vi "PNDT-Draw Line.vi"(0 "picture":picture, 2 "end point":cluster{"x":i16, "y":i16}, 3 "absolute coordinates?(T)":bool=TRUE, 4 "pen":T1={"Lable"="", "Visible"=FALSE, "Width"=1, "Colour"=10263708, "Line"=enum."DashDotDot"} {"Width" min=1 max=5}) -> (6 "new picture":picture)   [LabVIEW 2026, in "MicroPulse_Driver.lvlib"]
doc: "Draws a line from the current pen position to the specified location in a picture."
uses:
  MicroPulse_Driver.lvlib
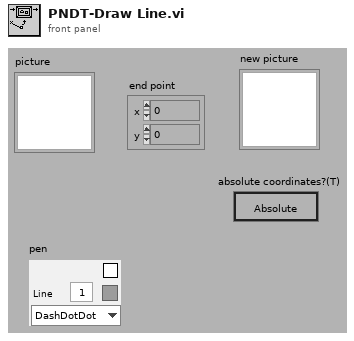
[diagram p1: front panel]
types:
  T1 = cluster{"Lable":string, "Visible":bool, "Width":u16, "Colour":u32, "Line":enum32{"Solid", "Dash", "Dot", "DashDot", "DashDotDot"}}
  T2 = enum32{"Solid", "Dash", "Dot", "DashDot", "DashDotDot"}
  T3 = cluster{"opcode-Select Pen":i16, "size":i32, "PictPen ID":i32, "pen mask":i32, "Colour":u32, "Width":u16, "Line":enum32{"Solid", "Dash", "Dot", "DashDot", "DashDotDot"}}
  T4 = cluster{"opcode-Line":i16, "size":i32, cluster{"y":i16, "x":i16}}
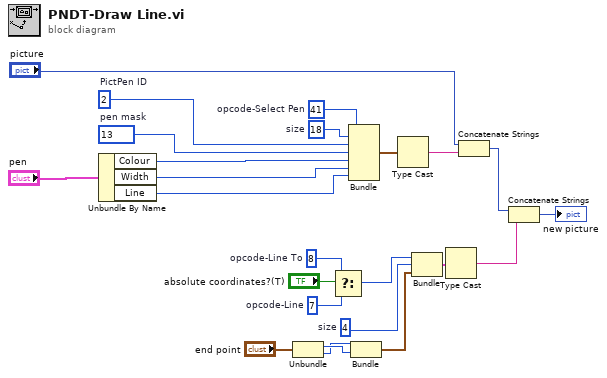
[diagram p0: block diagram]
diagram:
  w7 = 13  # pen mask
  w8 = 2  # PictPen ID
  w11 = i16 41  # opcode-Select Pen
  w10 = 18  # size
  w22 = i16 7  # opcode-Line
  w23 = i16 8  # opcode-Line To
  w20 = 4  # size
  n1 = Unbundle By Name("pen") -> ("Colour"=w4:u32, "Width"=w6:u16, "Line"=w5:T2)
  n2 = Unbundle("end point") -> ("x"=w16:i16, "y"=w15:i16)
  n3 = Select(t=w23, s="absolute coordinates?(T)", f=w22) -> (s? t:f=w21:i16)
  n4 = Bundle("opcode-Select Pen"=w11, "size"=w10, "PictPen ID"=w8, "pen mask"=w7, "Colour"=w4, "Width"=w6, "Line"=w5) -> (w9:T3)  [unwired: 1 in]
  n5 = Bundle("y"=w15, "x"=w16) -> (w14:cluster{"y":i16, "x":i16})  [unwired: 1 in]
  n6 = Type Cast(x=w9) -> (*(type *) &x=w12:string)  [unwired: 1 in]
  n7 = Bundle("opcode-Line"=w21, "size"=w20, w14) -> (w18:T4)  [unwired: 1 in]
  n8 = Type Cast(x=w18) -> (*(type *) &x=w17:string)  [unwired: 1 in]
  n9 = Concatenate Strings("picture", w12) -> (w3:picture)
  n10 = Concatenate Strings(w3, w17) -> (→"new picture":picture)
